vi "libssh2_userauth_banner.vi"(8 "error in (no error)":errorcluster, 11 "session":T1) -> (0 "error out":errorcluster, 2 "banner":string)   [LabVIEW 2013, in "libssh2.lvlib"]
doc: "Gets the server's userauth banner message."
uses:
  libssh2.lvlib
  Session Refnum.ctl
  Not A Session.vi
  <vilib>/Utility/error.llb/Error Cluster From Error Code.vi
  Global Settings.vi
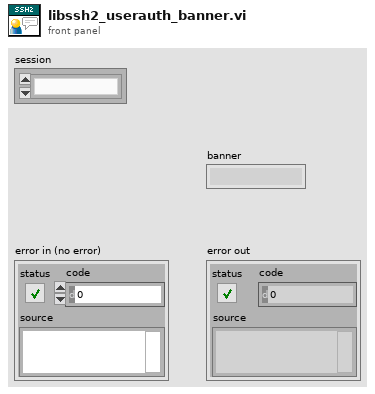
[diagram p1: front panel]
types:
  T1 = typedef "libssh2.lvlib/Session Refnum.ctl" = refnum<k1>
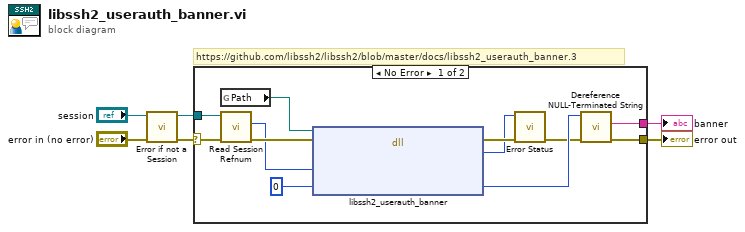
[diagram p0: block diagram]
diagram:
  # "https://github.com/libssh2/libssh2/blob/master/docs/libssh2_userauth_banner.3"
  n1 = call "Error if not a Session.vi"("error in (no error)"="error in (no error)", "session"="session") -> ("error out"=w3:errorcluster, "session out"=w1:T1)  [unwired: 8 in]
  n2 = case shown="No Error" w3 {
    selector: w3 -> [w13 w19]
    tunnel: [w10 w19] -> w6
    tunnel: [w17 _] -> w5
    tunnel: w1 -> [w15 _]
    frame No Error {
      n3 = global read "Global Settings.vi" "Path"() -> (w9:path)
      n4 = call "Read Session Refnum.vi"("error in (no error)"=w13, "session"=w15) -> ("error out"=w16:errorcluster, "LIBSSH2_SESSION*"=w14:u64)  [unwired: 8 in]
      n5 = dll-call lib="C:/Users/pasca/source/repos/libssh2-labview/libssh2/libssh2**.*" fn="libssh2_userauth_banner"(path in=w9, error in=w16, "session"=w14, "banner"=u64 0) -> (error out=w11:errorcluster, "return value"=w7:i32, "banner"=w12:u64)  [unwired: 2 in, 1 out]
      n6 = call "Error Status.vi"("error in (no error)"=w11, "return value"=w7) -> ("error out"=w8:errorcluster)  [unwired: 8 in, 1 out]
      n7 = call "Dereference NULL-Terminated String.vi"("error in (no error)"=w8, "char*"=w12) -> ("error out"=w10:errorcluster, "string"=w17:string)  [unwired: 8 in]
    }
    frame Error {
    }
  }
  "error out" <- w6
  "banner" <- w5
